vi "Set Relay.vi"(0 "connection ID":refnum<k16>, 1 "address":u32, 2 "port":u16, 5 "Relay Number":u16, 7 "Relay State":T1 items=["LOW", "HIGH"], 9 "timeout ms (1000)":i32=1000, 11 "error in (no error)":errorcluster, 12 "mask":u16) -> (4 "connection ID out":refnum<k16>, 6 "received data":string, 15 "error out":errorcluster)   [LabVIEW 2016, in "instr.lvlib"]
doc: "Sets given relay to given state."
uses:
  instr.lvlib
  IO State.ctl
panel:
  out "Send String":string
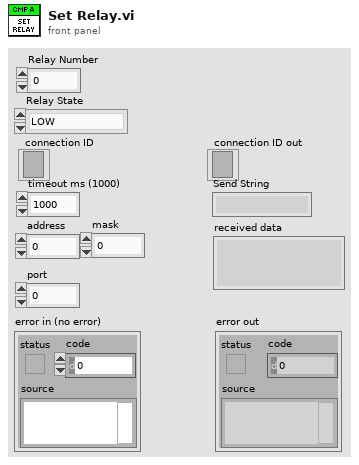
[diagram p1: front panel]
types:
  T1 = typedef "instr.lvlib/IO State.ctl" = u16
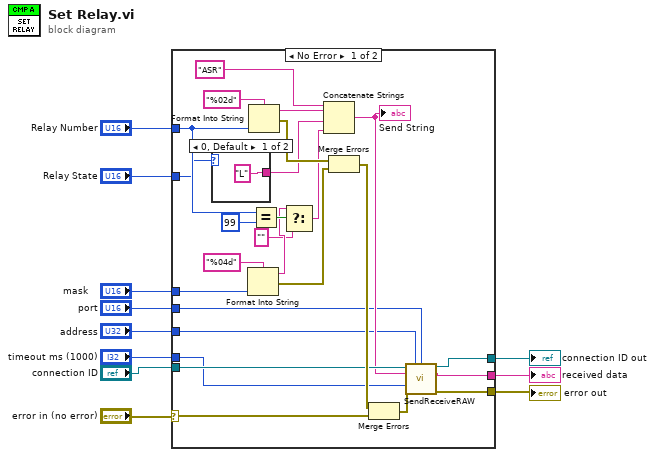
[diagram p0: block diagram]
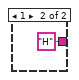
[diagram p2: hidden frame]
diagram:
  n1 = case shown="No Error" "error in (no error)" {
    selector: "error in (no error)" -> [w34 w41]
    tunnel: [w31 w41] -> w11
    tunnel: [w30 _] -> w9
    tunnel: "timeout ms (1000)" -> [w26 _]
    tunnel: "connection ID" -> [w28 w40]
    tunnel: [w29 w40] -> w6
    tunnel: "Relay Number" -> [w20 _]
    tunnel: "Relay State" -> [w13 _]
    tunnel: "address" -> [w24 _]
    tunnel: "port" -> [w23 _]
    tunnel: "mask" -> [w21 _]
    frame No Error {
      n2 = case shown="0, Default" w13 {
        tunnel: ["L" "H"] -> w14
        frame 0, Default {
        }
        frame 1 {
        }
      }
      n3 = Format Into String(format string="%04d", w21) -> (resulting string=w17:string, error out=w12:errorcluster)  [unwired: 2 in]
      n4 = Format Into String(format string="%02d", w20) -> (resulting string=w32:string, error out=w35:errorcluster)  [unwired: 2 in]
      n5 = Equal?(x=w20, y=u16 99) -> (x = y?=w18:bool)
      n6 = Select(t=w17, s=w18, f="") -> (s? t:f=w15:string)
      n7 = Concatenate Strings("ASR" ("data in"), w32, w14, w15) -> (w25:string)
      "Send String" <- w25
      n8 = Merge Errors(w35, w12) -> (w33:errorcluster)
      n9 = Merge Errors(w33, w34) -> (w27:errorcluster)
      n10 = call "SendReceiveRAW.vi"("connection ID"=w28, "address"=w24, "port"=w23, "RAW data in"=w25, "timeout ms (1000)"=w26, "error in (no error)"=w27) -> ("connection ID out"=w29:refnum<k16>, "received data"=w30:string, "error out"=w31:errorcluster)  [unwired: 7 in]
    }
    frame Error {
    }
  }
  "error out" <- w11
  "received data" <- w9
  "connection ID out" <- w6
